vi "Set Fix Operation Set Point.vi"(8 "error in":errorcluster, 10 "Set Point":dbl, 11 "VISA resource name":refnum<visa-resource-name>) -> (0 "error out":errorcluster, 2 "Successfully":bool, 3 "VISA resource name out":refnum<visa-resource-name>)   [LabVIEW 2016, in "Samwontech TEMP2xxx.lvlib"]
doc: "Set FIX operation Set Point \nD-Register D104 (FIX.TSP)"
uses:
  <instrlib>/Samwontech TEMP2xxx/Samwontech TEMP2xxx.lvlib
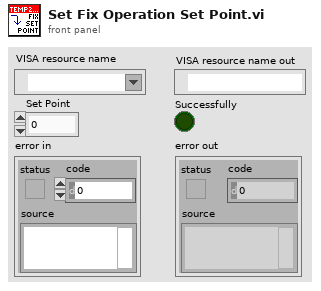
[diagram p1: front panel]
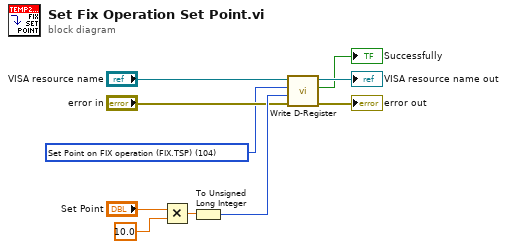
[diagram p0: block diagram]
diagram:
  w3 = u32 104 items=["Current PV (NPV)"=1, "Operation Control (COM.OPMODE)"=102, "Set Point on FIX operation (FIX.TSP)"=104, "Operation Mode (OP.MODE)"=106] ("D-Registers Map")
  n1 = Multiply(x="Set Point", y=10.0) -> (x*y=w8:dbl)
  n2 = To Unsigned Long Integer(number=w8) -> (unsigned 32bit integer=w7:u32)
  n3 = call <instrlib>:"Write D-Register.vi"("error in"="error in", "Data"=w7, "D-register number"=w3, "VISA resource name"="VISA resource name") -> ("error out"=→"error out":errorcluster, "Successfully"=→"Successfully":bool, "VISA resource name out"=→"VISA resource name out":refnum<visa-resource-name>)  [unwired: 4 in, 1 out]
